vi "Write to File.vi"() -> ()   [LabVIEW 2013]
uses:
  <vilib>/Utility/file.llb/Write To Spreadsheet File (DBL).vi
  <vilib>/Utility/file.llb/Read From Spreadsheet File (DBL).vi
panel:
  out "x+1":dbl
  out "Path":string
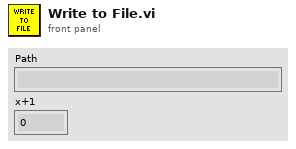
[diagram p1: front panel]
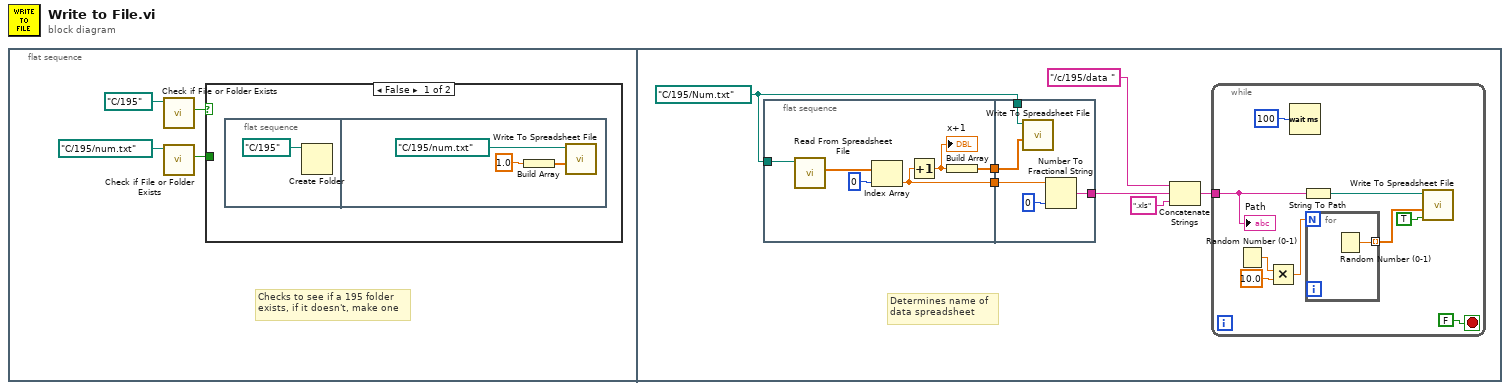
[diagram p0: block diagram]
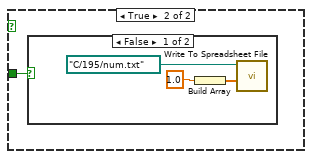
[diagram p2: hidden frame]
diagram:
  n1 = flat-sequence {
    frame #0 {
      # "Checks to see if a 195 folder\nexists, if it doesn't, make one"
      n2 = call <vilib>:"Check if File or Folder Exists.vi"("path"=path "C:/195") -> ("file or folder exists?"=w2:bool)  [unwired: 8 in, 2 out]
      n3 = call <vilib>:"Check if File or Folder Exists.vi"("path"=path "C:/195/num.txt") -> ("file or folder exists?"=w1:bool)  [unwired: 8 in, 2 out]
      n4 = case shown="False" w2 {
        tunnel: w1 -> [_ w9]
        frame False {
          n5 = flat-sequence {
            frame #0 {
              n6 = Create Folder(path (use dialog)=path "C:/195") -> ()  [unwired: 2 in, 3 out]
            }
            frame #1 {
              n7 = Build Array(1.0 ("element")) -> (w7:dbl[])
              n8 = call-poly <vilib>:"Write To Spreadsheet File.vi"("1D data"=w7, "file path (dialog if empty)"=path "C:/195/num.txt") -> ()  [unwired: 6 in, 1 out]
            }
          }
        }
        frame True {
          n9 = case shown="False" w9 {
            frame False {
              n10 = Build Array(1.0 ("element")) -> (w11:dbl[])
              n11 = call-poly <vilib>:"Write To Spreadsheet File.vi"("1D data"=w11, "file path (dialog if empty)"=path "C:/195/num.txt") -> ()  [unwired: 6 in, 1 out]
            }
            frame True {
            }
          }
        }
      }
    }
    frame #1 {
      w14 = path "C:/195/Num.txt" ("file path (use dialog)")
      # "Determines name of\ndata spreadsheet"
      n12 = flat-sequence {
        tunnel: w14 -> [w21]
        tunnel: [w22] -> w19
        tunnel: [w20] -> w18
        tunnel: w19 -> [w30]
        tunnel: w14 -> [w29]
        tunnel: w18 -> [w28]
        tunnel: [w26] -> w13
        frame #0 {
          n13 = call-poly <vilib>:"Read From Spreadsheet File.vi"("file path (dialog if empty)"=w21) -> ("first row"=w24:dbl[])  [unwired: 6 in, 4 out]
          n14 = Index Array(array=w24, index=0) -> (element=w20:dbl)
          n15 = Increment(x=w20) -> (x+1=w23:dbl)
          "x+1" <- w23
          n16 = Build Array(w23) -> (w22:dbl[])
        }
        frame #1 {
          n17 = call-poly <vilib>:"Write To Spreadsheet File.vi"("1D data"=w30, "file path (dialog if empty)"=w29) -> ()  [unwired: 6 in, 1 out]
          n18 = Number To Fractional String(number=w28, precision (6)=i16 0) -> (F-format string=w26:string)  [unwired: 2 in]
        }
      }
      n19 = Concatenate Strings("/c/195/data ", w13, ".xls" ("string")) -> (w15:string)
      n20 = while {
        tunnel: w15 -> [w31]
        stop <- FALSE stop-if-true
        n21 = Random Number (0-1)() -> (number: 0 to 1=w37:dbl)
        n22 = Multiply(x=w37, y=10.0) -> (x*y=w35:dbl)
        n23 = Wait (ms)(milliseconds to wait=u32 100) -> ()  [unwired: 1 out]
        n24 = String To Path(string=w31) -> (path=w33:path)
        n25 = for {
          N: w35 -> [_]
          tunnel: [w40] -> w34 mode=indexing
          n26 = Random Number (0-1)() -> (number: 0 to 1=w40:dbl)
        }
        n27 = call-poly <vilib>:"Write To Spreadsheet File.vi"("append to file? (new file:F)"=TRUE, "1D data"=w34, "file path (dialog if empty)"=w33) -> ()  [unwired: 5 in, 1 out]
        "Path" <- w31
      }
    }
  }
